vi "ICM Editor Stop.vi"() -> ()   [LabVIEW 2018]
panel:
  in  "Stop":bool
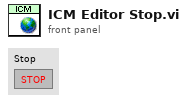
[diagram p1: front panel]
diagram:
